vi "全站仪通信.vi"() -> ()   [LabVIEW 2016]
uses:
  <vilib>/Instr/_visa.llb/VISA Configure Serial Port (Instr).vi
panel:
  out "XY图":cluster{dbl[], dbl[]}(graph)
  in  "开始坐标发送":bool
  out "接收区":string
  in  "流控制":u32
  in  "停止位":u32=1
  in  "奇偶校验":u32
  in  "数据比特":u32=8
  in  "波特率":u32=9600
  in  "流控制":u32
  in  "停止位":u32=1
  in  "奇偶校验":u32
  in  "数据比特":u32=8
  in  "波特率":u32=9600
  in  "输出串口":refnum<visa-resource-name>="COM1"
  in  "输入串口":refnum<visa-resource-name>="COM1"
  in  "stop":bool
  in  "OK Button":bool
  in  "发送区":string
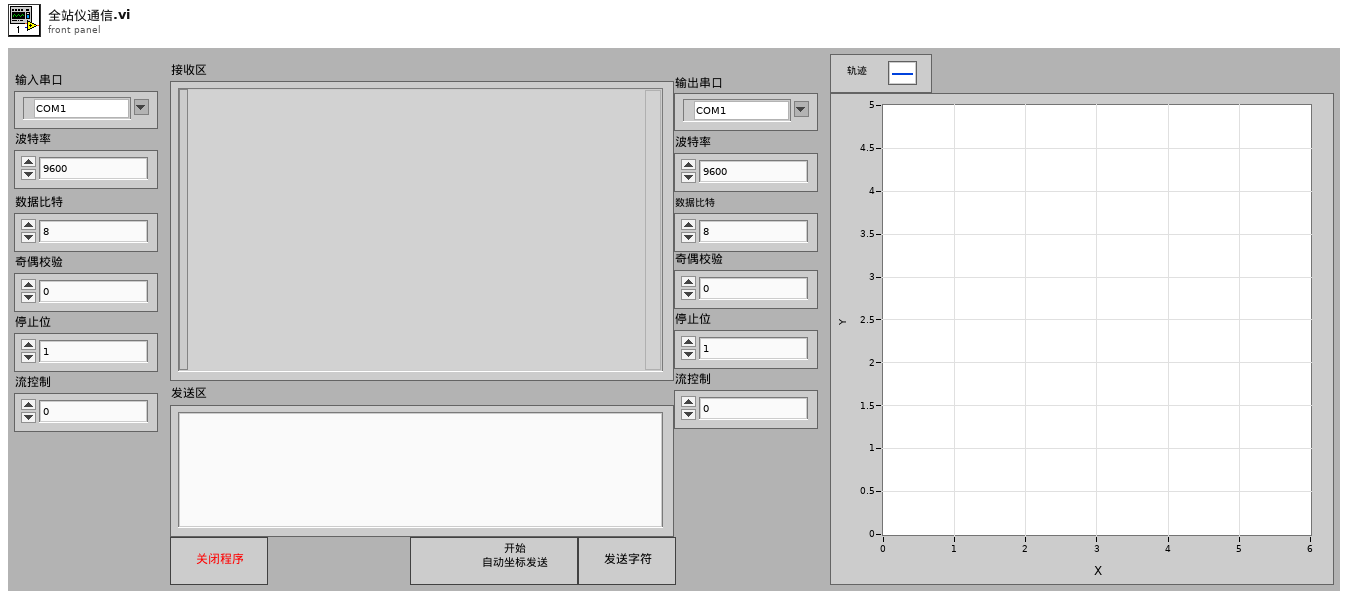
[diagram p1: front panel]
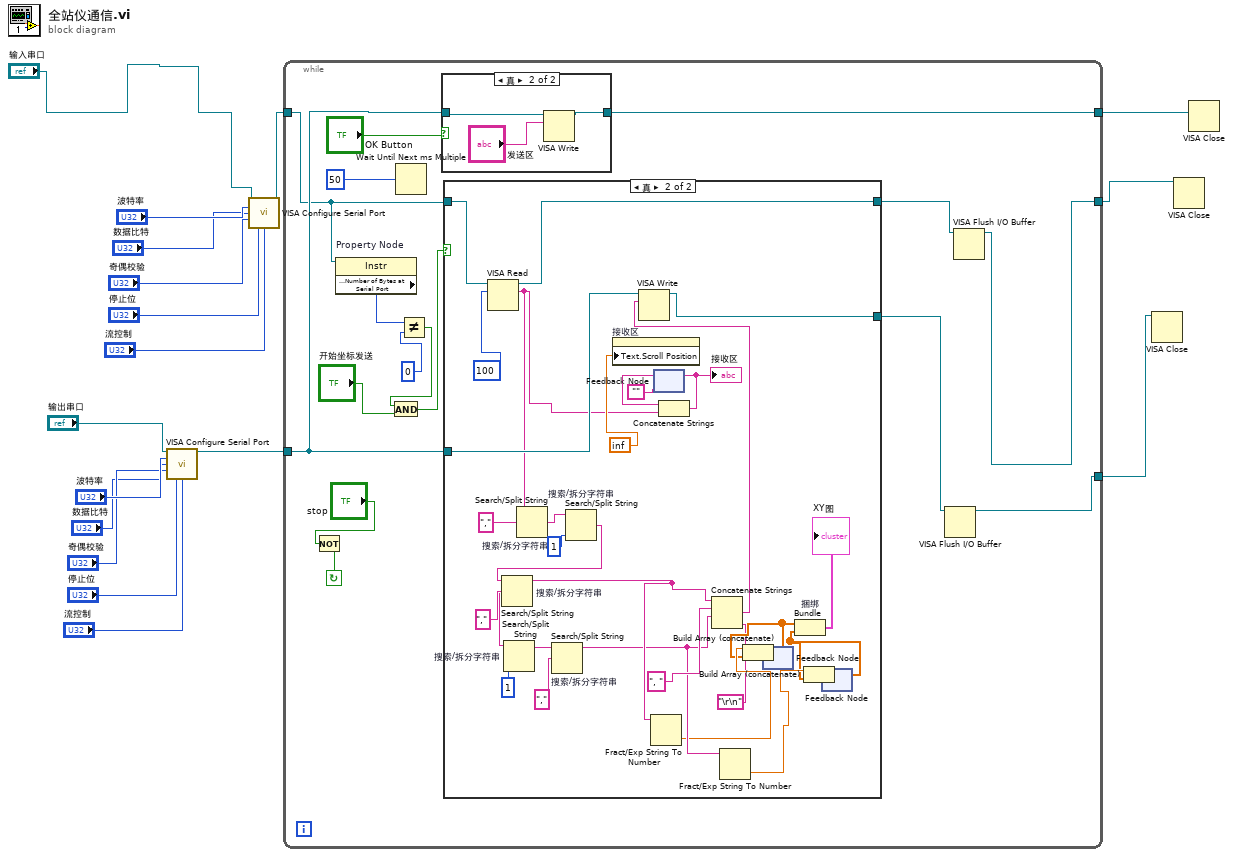
[diagram p0: block diagram]
diagram:
  n1 = call-poly "VISA Configure Serial Port"("VISA resource name"="输出串口", "baud rate (9600)"="波特率", "data bits (8)"="数据比特", "parity (0:none)"="奇偶校验", "stop bits (10: 1 bit)"="停止位", "flow control (0:none)"="流控制") -> ("VISA resource name out"=w16:refnum<visa-resource-name>)  [unwired: 1 in, 8 out]
  n2 = call-poly "VISA Configure Serial Port"("VISA resource name"="输入串口", "baud rate (9600)"="波特率", "data bits (8)"="数据比特", "parity (0:none)"="奇偶校验", "stop bits (10: 1 bit)"="停止位", "flow control (0:none)"="流控制") -> ("VISA resource name out"=w4:refnum<visa-resource-name>)  [unwired: 1 in, 8 out]
  n3 = while {
    tunnel: w4 -> [w23]
    tunnel: [w32] -> w17
    tunnel: [w24] -> w2
    tunnel: w16 -> [w31]
    tunnel: [w26] -> w1
    stop <- w28 continue-if-true
    n4 = Not(x="stop") -> (.not. x?=w28:bool)
    n5 = property on="Property Node" class="Instr"(reference=w23) -> ("Serial Settings:Number of Bytes at Serial Port"=w22:u32)  [unwired: 1 in, 2 out]
    n6 = Wait Until Next ms Multiple(millisecond multiple=50) -> ()  [unwired: 1 out]
    n7 = Not Equal?(x=w22, y=0) -> (x != y?=w20:bool)
    n8 = And(x=w20, y="开始坐标发送") -> (x .and. y?=w18:bool)
    n9 = case shown="真" "OK Button" {
      tunnel: w31 -> [w67 w70]
      tunnel: [w67 w69] -> w32
      frame False {
      }
      frame True {
        n10 = VISA Write(VISA resource name=w70, write buffer="发送区") -> (VISA resource name out=w69:refnum<visa-resource-name>)  [unwired: 1 in, 2 out]
      }
    }
    n11 = case shown="真" w18 {
      tunnel: w23 -> [w35 w59]
      tunnel: [w35 w66] -> w25
      tunnel: w31 -> [w34 w65]
      tunnel: [w34 w62] -> w27
      frame False {
      }
      frame True {
        n12 = VISA Read(VISA resource name=w59, byte count=100) -> (VISA resource name out=w66:refnum<visa-resource-name>, read buffer=w48:string)  [unwired: 1 in, 2 out]
        n13 = Search/Split String "搜索/拆分字符串"(string=w48, search string/char (-)=",") -> (match + rest of string=w56:string)  [unwired: 3 out]
        n14 = Search/Split String "搜索/拆分字符串"(string=w56, offset (0)=1) -> (match + rest of string=w54:string)  [unwired: 1 in, 2 out]
        n15 = Search/Split String "搜索/拆分字符串"(string=w54, search string/char (-)=",") -> (substring before match=w45:string, match + rest of string=w52:string)  [unwired: 2 out]
        n16 = Search/Split String "搜索/拆分字符串"(string=w52, offset (0)=1) -> (match + rest of string=w50:string)  [unwired: 1 in, 2 out]
        n17 = Search/Split String "搜索/拆分字符串"(string=w50, search string/char (-)=",") -> (substring before match=w44:string)  [unwired: 3 out]
        n18 = property on="接收区" class="Str"("Text.Scroll Position"=inf) -> ()  [unwired: 2 in, 2 out]
        n19 = Fract/Exp String To Number(string=w45) -> (number=w41:dbl)  [unwired: 3 in, 1 out]
        n20 = feedback #1("") -> (w64:string)
        n21 = Concatenate Strings(w64, w48) -> (w61:string)
        "接收区" <- w61
        n22 = feedback-in #1(w61) -> ()
        n23 = Concatenate Strings(w45, ", " ("search string/char (-)"), w44, "\r\n") -> (w47:string)
        n24 = VISA Write(VISA resource name=w65, write buffer=w47) -> (VISA resource name out=w62:refnum<visa-resource-name>)  [unwired: 1 in, 2 out]
        n25 = Fract/Exp String To Number(string=w44) -> (number=w42:dbl)  [unwired: 3 in, 1 out]
        n26 = feedback #2() -> (w39:dbl[])  [unwired: 1 in]
        n27 = Build Array (concatenate)(w41, w39) -> (w40:dbl[])
        n28 = feedback-in #2(w40) -> ()
        n29 = feedback #3() -> (w37:dbl[])  [unwired: 1 in]
        n30 = Bundle "捆绑"(w39, w37) -> (→"XY图":cluster{dbl[], dbl[]})  [unwired: 1 in]
        n31 = Build Array (concatenate)(w42, w37) -> (w38:dbl[])
        n32 = feedback-in #3(w38) -> ()
      }
    }
    n33 = VISA Flush I/O Buffer(VISA resource name=w27) -> (VISA resource name out=w26:refnum<visa-resource-name>)  [unwired: 2 in, 1 out]
    n34 = VISA Flush I/O Buffer(VISA resource name=w25) -> (VISA resource name out=w24:refnum<visa-resource-name>)  [unwired: 2 in, 1 out]
  }
  n35 = VISA Close(VISA resource name=w1) -> ()  [unwired: 1 in, 1 out]
  n36 = VISA Close(VISA resource name=w2) -> ()  [unwired: 1 in, 1 out]
  n37 = VISA Close(VISA resource name=w17) -> ()  [unwired: 1 in, 1 out]
